vi "Remove JSON Tag.vi"(11 "Name":string) -> (2 "tagged as JSON text":bool, 3 "Name (tag stripped)":string)   [LabVIEW 2017, in "JSONtext.lvlib"]
uses:
  JSONtext.lvlib
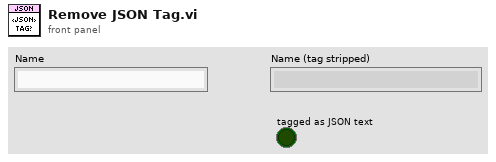
[diagram p1: front panel]
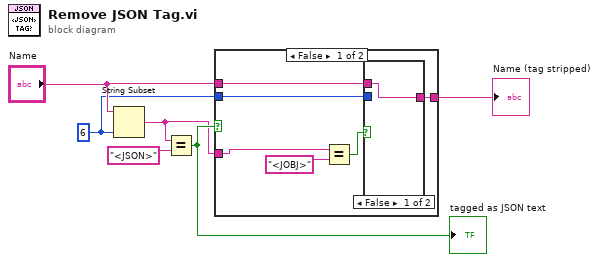
[diagram p0: block diagram]
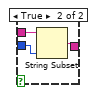
[diagram p2: hidden frame]
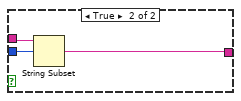
[diagram p3: hidden frame]
diagram:
  w2 = 6 ("length (rest)")
  n1 = String Subset(string="Name", length (rest)=w2) -> (substring=w1:string)  [unwired: 1 in]
  n2 = Equal?(x=w1, y="<JSON>") -> (x = y?=w6:bool)
  "tagged as JSON text" <- w6
  n3 = case shown="False" w6 {
    tunnel: [w9 w18] -> w4
    tunnel: "Name" -> [w10 w19]
    tunnel: w2 -> [w8 w17]
    tunnel: w1 -> [w11 _]
    frame False {
      n4 = Equal?(x=w11, y="<JOBJ>") -> (x = y?=w7:bool)
      n5 = case shown="False" w7 {
        tunnel: w10 -> [w13 w16]
        tunnel: [w13 w15] -> w9
        tunnel: w8 -> [_ w14]
        frame False {
        }
        frame True {
          n6 = String Subset(string=w16, length (rest)=w14) -> (substring=w15:string)  [unwired: 1 in]
        }
      }
    }
    frame True {
      n7 = String Subset(string=w19, offset (0)=w17) -> (substring=w18:string)  [unwired: 1 in]
    }
  }
  "Name (tag stripped)" <- w4
